vi "NI VeriStand - Get Macro Player State.vi"(8 "error in (no error)":errorcluster, 11 "MacroPlayer in":T2) -> (0 "error out":errorcluster, 2 "PlayState":T1, 3 "MacroPlayer out":T2)   [LabVIEW 2020, in "NI_VS MacroPlayerAPI.lvlib"]
doc: "Returns the current state of the Macro Player tool."
uses:
  <vilib>/NI VeriStand/Execution/MacroPlayer/NI_VS MacroPlayerAPI.lvlib
  <vilib>/NI VeriStand/Execution/MacroPlayer/MacroPlayerAPI.ctl
  NationalInstruments.VeriStand.ClientAPI
  <vilib>/NI VeriStand/Execution/MacroPlayer/Play State.ctl
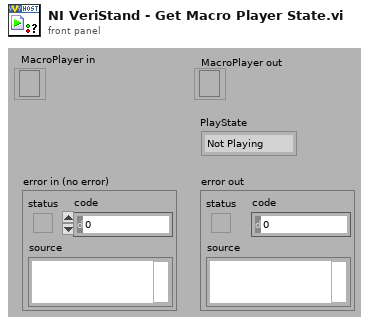
[diagram p1: front panel]
types:
  T1 = typedef "NI_VS MacroPlayerAPI.lvlib/Play State.ctl" = enum8{"Not Playing", "Playing", "Paused"}
  T2 = typedef "NI_VS MacroPlayerAPI.lvlib/MacroPlayerAPI.ctl" = refnum<k24>
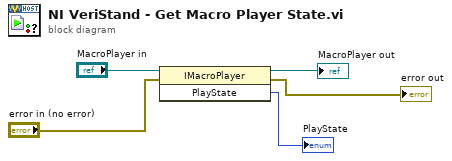
[diagram p0: block diagram]
diagram:
  n1 = invoke class="IMacroPlayer" method="PlayState"(reference="MacroPlayer in", error in="error in (no error)") -> (reference out=→"MacroPlayer out":T2, error out=→"error out":errorcluster, "PlayState"=→"PlayState":u8)  [unwired: 1 in]
